vi "Host.vi"() -> ()   [LabVIEW 2019]
panel:
  in  "stop":bool
  out "Load torque":dbl
  out "Duty cycle":dbl
  in  "Load torque":dbl
  in  "Duty cycle":dbl
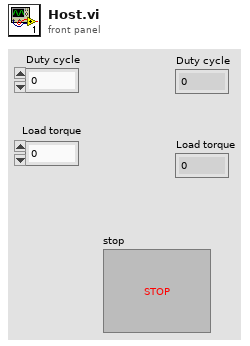
[diagram p1: front panel]
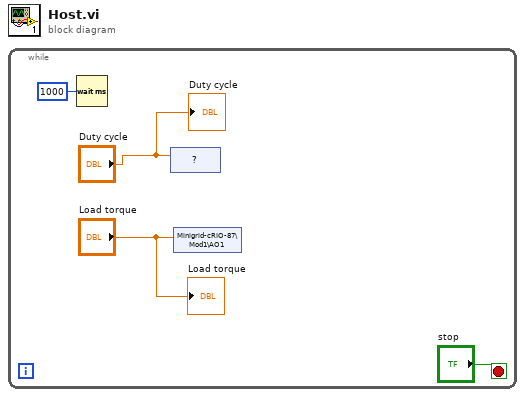
[diagram p0: block diagram]
diagram:
  n1 = while {
    stop <- "stop" stop-if-true
    n2 = Wait (ms)(milliseconds to wait=u32 1000) -> ()  [unwired: 1 out]
    n3 = shared-variable "?"("Duty cycle") -> ()  [unwired: 1 in, 1 out]
    n4 = shared-variable "Minigrid-cRIO-87\\Mod1\\AO1"("Load torque") -> ()  [unwired: 1 in, 1 out]
    "Duty cycle" <- "Duty cycle"
    "Load torque" <- "Load torque"
  }
